vi "Close.vi"(8 "error in (no error)":errorcluster, 11 "SSE Client in":refnum<class "SSE Client.lvclass">) -> (0 "error out":errorcluster)   [LabVIEW 2020, in "HTTP Server.lvlib" / "SSE Client.lvclass"]
uses:
  SSE Client.lvclass
  SSE Client.lvclass/SSE Client.ctl
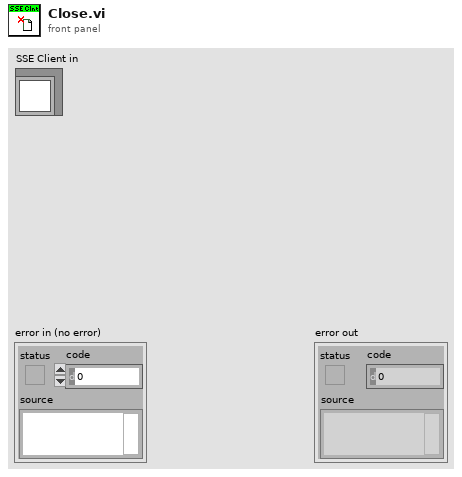
[diagram p1: front panel]
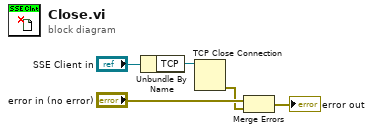
[diagram p0: block diagram]
diagram:
  n1 = Unbundle By Name("SSE Client in") -> ("TCP"=w3:refnum<k5>)
  n2 = TCP Close Connection(connection ID=w3) -> (error out=w1:errorcluster)  [unwired: 2 in, 1 out]
  n3 = Merge Errors("error in (no error)", w1) -> (→"error out":errorcluster)
